vi "phase_correct_coupling.vi"(4 "Really correct?":bool=TRUE, 6 "Is low?":bool, 10 "Complex coupling":cdb[][](array[numeric]) format="%#.3f", 11 "Ref carrier ampl":cdb[][][](array[numeric]) format="%#.3f") -> (2 "Phase corrected coupling":cdb[][](array[numeric]) format="%#.3f", 3 "Phase mismatch":dbl[][](array[numeric]) format="%#.3f")   [LabVIEW 2014]
panel:
  out "Ref magnitude":dbl[][](array[numeric]) format="%#.3f"
  out "Ref phase":dbl[][](array[numeric]) format="%#.3f"
  # "Is this a low rate coupling?"
  # "If false, don't actually do anything, just pass coupling through."
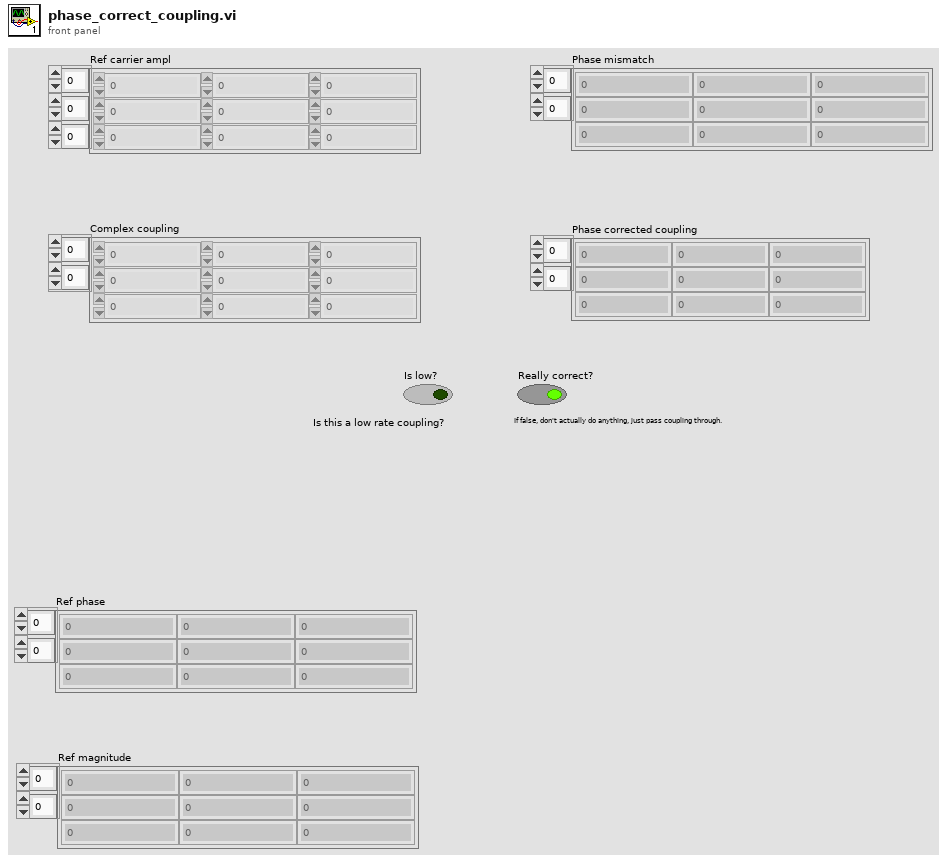
[diagram p1: front panel]
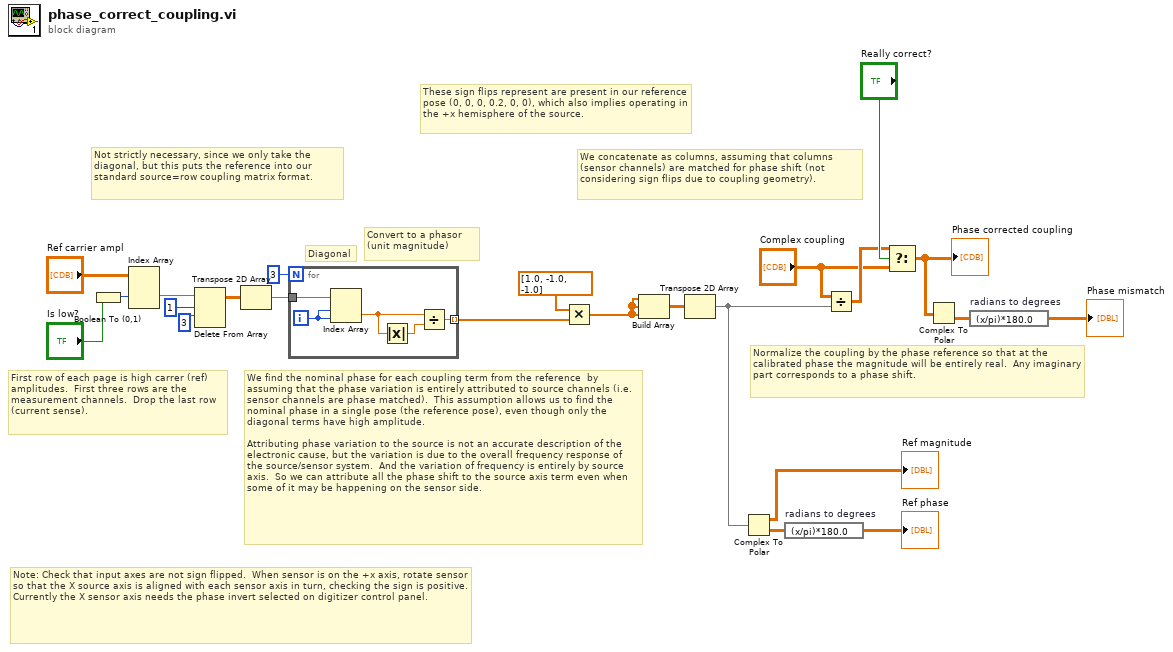
[diagram p0: block diagram]
diagram:
  # "Note: Check that input axes are not sign flipped.  When sensor is on the +x axis, rotate sensor so that the X source axis is aligned with each sensor axis in turn, checking the sign is positive.  Currently the X sensor axis needs the phase invert selected on digitizer control panel."
  # "These sign flips represent are present in our reference pose (0, 0, 0, 0.2, 0, 0), which also implies operating in the +x hemisphere of the source."
  # "Normalize the coupling by the phase reference so that at the calibrated phase the magnitude will be entirely real.  Any imaginary part corresponds to a phase shift."
  # "Not strictly necessary, since we only take the diagonal, but this puts the reference into our standard source=row coupling matrix format."
  # "We concatenate as columns, assuming that columns (sensor channels) are matched for phase shift (not considering sign flips due to coupling geometry)."
  # "Convert to a phasor (unit magnitude)"
  # "Diagonal"
  # "We find the nominal phase for each coupling term from the reference  by assuming that the phase variation is entirely attributed to source channels (i.e. sensor channels are phase matched).  This assumption allows us to find the nominal phase in a single pose (the reference pose), even though only the diagonal terms have high amplitude. \n\nAttributing phase variation to the source is not an accurate description of the electronic cause, but the variation is due to the overall frequency response of the source/sensor system.  And the variation of frequency is entirely by source axis.  So we can attribute all the phase shift to the source axis term even when some of it may be happening on the sensor side."
  # "First row of each page is high carrer (ref) amplitudes.  First three rows are the measurement channels.  Drop the last row (current sense)."
  n1 = Boolean To (0,1)(Boolean="Is low?") -> (0, 1=w16:i16)
  n2 = Index Array(array="Ref carrier ampl", index (dim 1)=w16) -> (element=w18:cdb[][])  [unwired: 2 in]
  n3 = Delete From Array(array=w18, length=1, index (row)=3) -> (array with subset deleted=w21:cdb[][])  [unwired: 1 in, 1 out]
  n4 = Transpose 2D Array(2D array=w21) -> (transposed array=w22:cdb[][])
  n5 = for {
    N: 3 -> [_]
    tunnel: w22 -> [w28]
    tunnel: [w24] -> w11 mode=indexing
    i -> [w27]
    n6 = Index Array(array=w28, index (row)=w27, index (col)=w27) -> (element=w25:cdb)
    n7 = Absolute Value(x=w25) -> (abs(x)=w26:dbl)
    n8 = Divide(x=w25, y=w26) -> (x/y=w24:cdb)
  }
  n9 = Multiply(x=dbl[] [1.0, -1.0, -1.0] ("Sign flips"), y=w11) -> (x*y=w8:cdb[])
  n10 = Build Array(w8, w8, w8) -> (w6:cdb[][])
  n11 = Transpose 2D Array(2D array=w6) -> (transposed array=w5:cdb[][])
  n12 = Complex To Polar(r * e^(i*theta)=w5) -> (r=→"Ref magnitude":dbl[][], theta=w9:dbl[][])
  n13 = expression code="(x/pi)*180.0" "radians to degrees"(w9) -> (→"Ref phase":dbl[][])
  n14 = Divide(x="Complex coupling", y=w5) -> (x/y=w3:cdb[][])
  n15 = Select(t=w3, s="Really correct?", f="Complex coupling") -> (s? t:f=w1:cdb[][])
  "Phase corrected coupling" <- w1
  n16 = Complex To Polar(r * e^(i*theta)=w1) -> (theta=w14:dbl[][])  [unwired: 1 out]
  n17 = expression code="(x/pi)*180.0" "radians to degrees"(w14) -> (→"Phase mismatch":dbl[][])
